vi "DisplayName.vi"(1 "State In":T1) -> (0 "Name":string)   [LabVIEW 2018, in "Foreign Key Sort.xnode"]
doc: "This ability is deprecated; prefer GetDisplayName2.\n\nThis ability VI is used to supply LabVIEW with the name of your XNode. This is used as the default value for the label, it is used to mark entries in the error list and the difference list.\n\nDefault behavior: None.\n\nThis ability does not provide UI and OS messages are not handled."
uses:
  Foreign Key Sort.xnode
  State.ctl
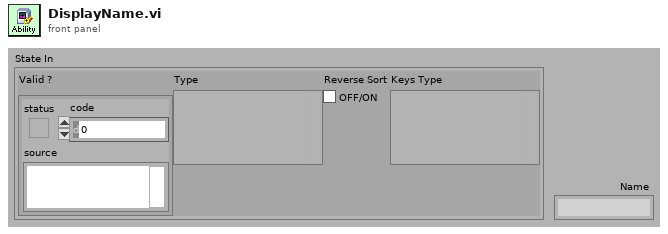
[diagram p1: front panel]
types:
  T1 = typedef "Foreign Key Sort.xnode/State.ctl" = cluster{"Valid ?":errorcluster, "Type":variant, "Reverse Sort":bool, "Keys Type":variant}
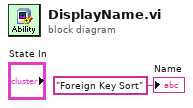
[diagram p0: block diagram]
diagram:
  "Name" <- "Foreign Key Sort" ("Name")
